vi "Setup UI.vi"(8 "error in (no error)":errorcluster, 10 "Set UI to input? (F)":bool, 11 "Wavelength Digikröm in":refnum<class "Wavelength Digikröm.lvclass">) -> (0 "error out":errorcluster, 3 "Wavelength Digikröm out":refnum<class "Wavelength Digikröm.lvclass">)   [LabVIEW 2009, in "Wavelength Digikröm.lvclass"]
doc: "Scanner::Setup is a constructor that has no parameters and faces the user. The Factory calls this VI to let the user configure this Scanner. It is dynamically dispatched in order to let the user choose the type as well as the options of the scanner."
uses:
  Wavelength Digikröm.lvclass
  Scanner/Scanner.lvclass
panel:
  # "Digikrom DK240 Setup"
  # "No options yet."
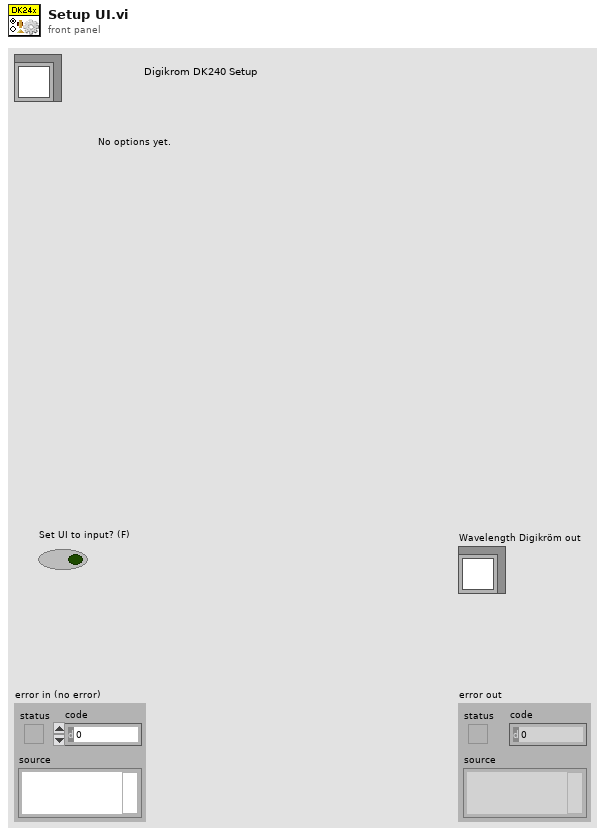
[diagram p1: front panel]
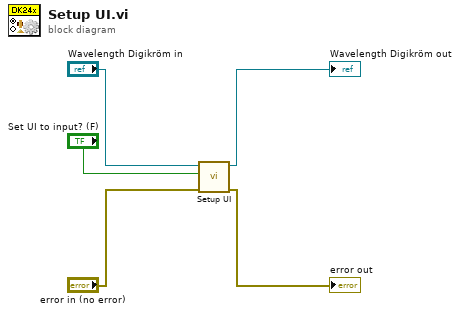
[diagram p0: block diagram]
diagram:
  n1 = call-parent "Setup UI.vi"("error in (no error)"="error in (no error)", "Set UI to input? (F)"="Set UI to input? (F)", "Scanner in"="Wavelength Digikröm in") -> ("error out"=→"error out":errorcluster, "Scanner out"=→"Wavelength Digikröm out":refnum<class "Wavelength Digikröm.lvclass">)  [unwired: 7 out]
